vi "default responder action.vi"(10 "dictionary":variant, 11 "standard input":string) -> (1 "code":u32, 2 "standard error":string, 3 "standard out":string)   [LabVIEW 2013]
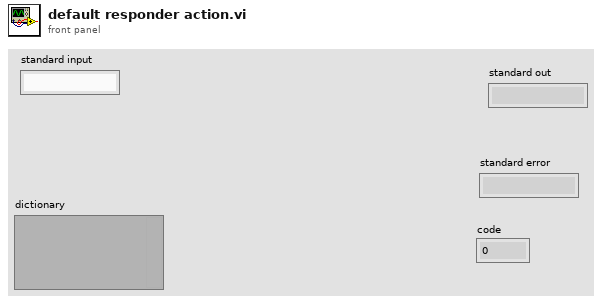
[diagram p1: front panel]
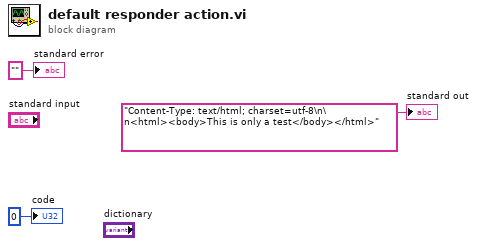
[diagram p0: block diagram]
diagram:
  "standard out" <- "Content-Type: text/html; charset=utf-8\n\n<html><body>This is only a test</body></html>" ("standard out")
  "standard error" <- "" ("standard error")
  "code" <- u32 0 ("code")
